vi "Close Contexts.vi"(8 "error in (no error)":errorcluster, 11 "Entity Editor in":refnum<class "Entity Editor.lvclass">) -> (0 "error out":errorcluster, 3 "Entity Editor out":refnum<class "Entity Editor.lvclass">)   [LabVIEW 2020, in "Conditum-Tools.lvlib" / "Entity Editor.lvclass"]
uses:
  Entity Editor.lvclass
  Context.ctl
  Conditum-Tools.lvlib
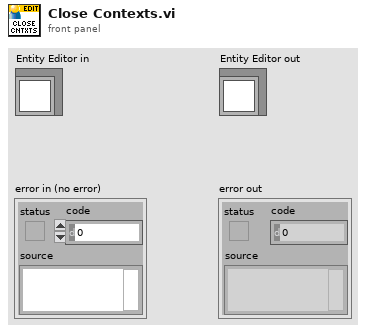
[diagram p1: front panel]
types:
  T1 = typedef "Conditum-Tools.lvlib/Context.ctl" = enum16{"Editor", "Entity"}
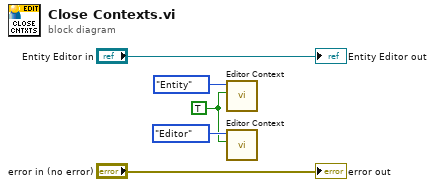
[diagram p0: block diagram]
diagram:
  w1 = TRUE ("Close (F)")
  n1 = call "Editor Context.vi"("Close (F)"=w1, "Context"=Context."Entity") -> ()  [unwired: 8 in, 2 out]
  n2 = call "Editor Context.vi"("Close (F)"=w1, "Context"=Context."Editor") -> ()  [unwired: 8 in, 2 out]
  "error out" <- "error in (no error)"
  "Entity Editor out" <- "Entity Editor in"
